vi "InstrQuery.vi"(8 "error in (no error)":errorcluster, 10 "Command string":string, 11 "InstControl in":refnum<class "InstrControl.lvclass">) -> (0 "error out":errorcluster, 2 "Instrument response":string, 3 "InstControl out":refnum<class "InstrControl.lvclass">)   [LabVIEW 2018, in "InstrControl.lvclass"]
uses:
  InstrControl.lvclass
  InstrControl.lvclass/InstrControl.ctl
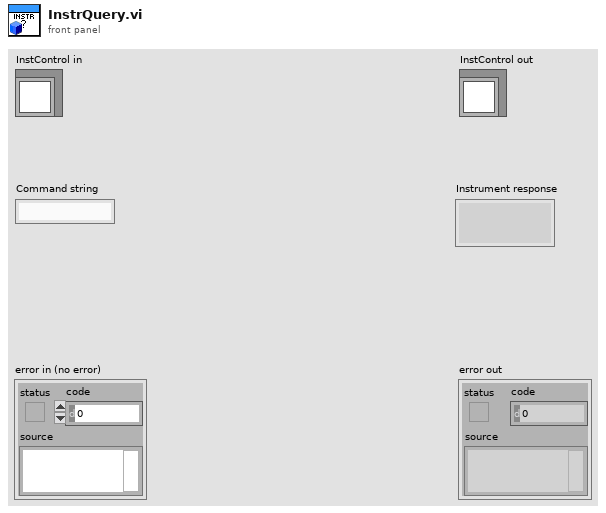
[diagram p1: front panel]
types:
  T1 = cluster{"error":bool, "code":i32, "source":string}
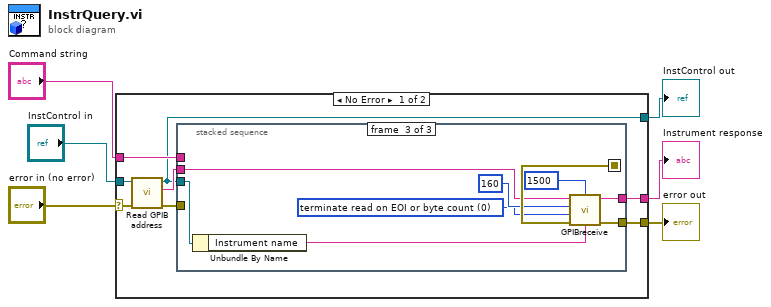
[diagram p0: block diagram]
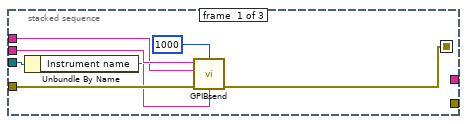
[diagram p2: hidden frame]
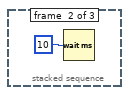
[diagram p3: hidden frame]
diagram:
  n1 = case shown="No Error" "error in (no error)" {
    selector: "error in (no error)" -> [w10 w33]
    tunnel: [w14 w33] -> w5
    tunnel: [w7 w32] -> w3
    tunnel: "InstControl in" -> [w12 w32]
    tunnel: "Command string" -> [w13 _]
    tunnel: [w8 _] -> w1
    frame No Error {
      n2 = call-dynamic "Read GPIB address.vi"("error in (no error)"=w10, "InstControl in"=w12) -> ("error out"=w9:errorcluster, "GPIB address"=w11:string, "InstControl out"=w7:refnum<class "InstrControl.lvclass">)  [unwired: 7 in]
      n3 = stacked-sequence {
        seq-local: [w18 _ _] -> [_ _ w30]
        tunnel: w11 -> [w21 _ w29]
        tunnel: w9 -> [w20 _ _]
        tunnel: [_ _ w31] -> w14
        tunnel: w13 -> [w19 _ _]
        tunnel: [_ _ w27] -> w8
        tunnel: w7 -> [w17 _ w26]
        frame #0 {
          n4 = Unbundle By Name(w17) -> ("Instrument name"=w16:string)
          n5 = call "GPIBsend.vi"("timeout ms"=u32 1000, "address string"=w21, "write buffer"=w19, "source"=w16, "error in"=w20) -> ("error out"=w18:errorcluster)  [unwired: 2 in, 2 out]
        }
        frame #1 {
          n6 = Wait (ms)(milliseconds to wait=10) -> ()  [unwired: 1 out]
        }
        frame #2 {
          w23 = 0 items=["terminate read on EOI or byte count", "terminate read on EOI, byte count, or CR", "terminate read on EOI, byte count, or LF"] ("read mode")
          n7 = Unbundle By Name(w26) -> ("Instrument name"=w25:string)
          n8 = call "GPIBreceive.vi"("timeout ms"=u32 1500, "address string"=w29, "byte count"=160, "source"=w25, "read mode"=w23, "error in"=w30) -> ("read buffer"=w27:string, "error out"=w31:T1)  [unwired: 1 in, 1 out]
        }
      }
    }
    frame Error {
    }
  }
  "error out" <- w5
  "InstControl out" <- w3
  "Instrument response" <- w1
